vi "nPoints Concept - Pushbutton.vi"() -> ()   [LabVIEW 2013]
uses:
  <vilib>/Utility/error.llb/DialogType.ctl
  <vilib>/DAQmx/read.llb/DAQmx Read (Digital 1D Bool 1Chan 1Samp).vi
  <vilib>/DAQmx/create/channels.llb/DAQmx Create Channel (DI-Digital Input).vi
  <vilib>/DAQmx/miscellaneous.llb/DAQmx Fill In Error Info.vi
panel:
  out "Digital Data":i16(graph)
  in  "Line(s)":tag="Dev1/port0/line0:7"
  in  "Stop":bool
  out "Blank Button":bool
  # "Pushbutton Switch"
  # "5V"
  # "DIO"
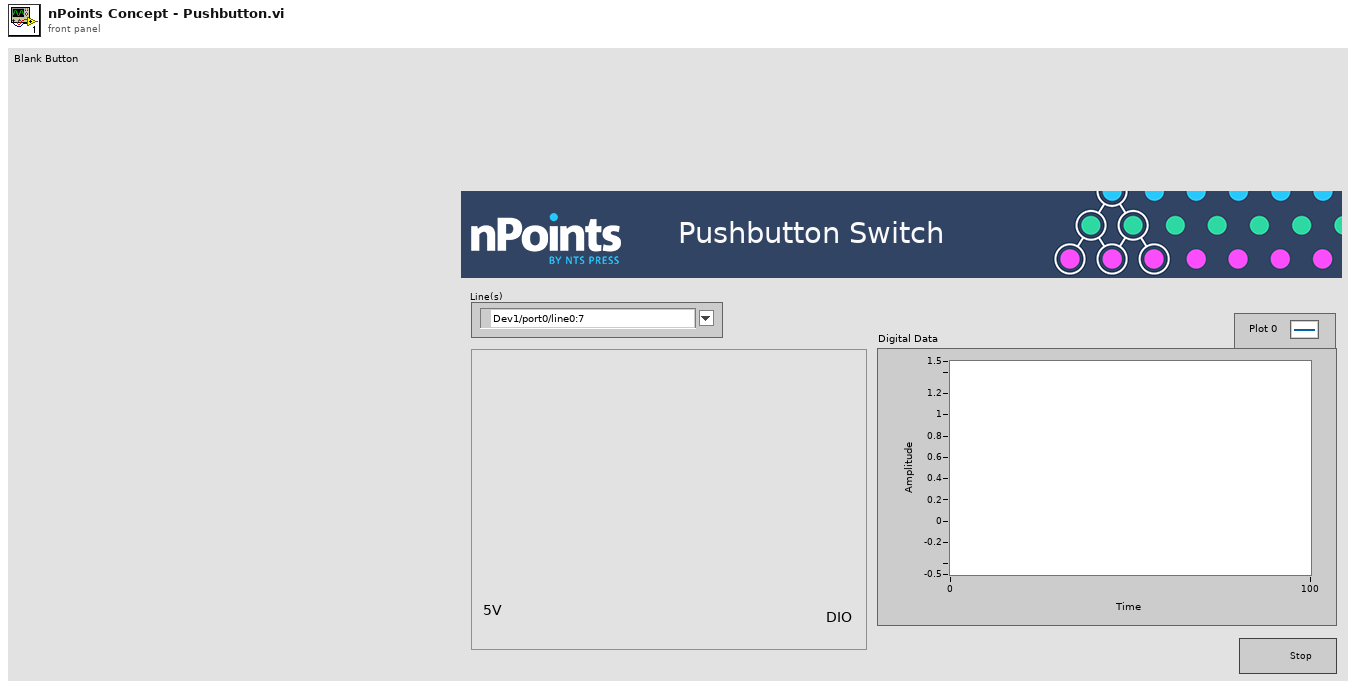
[diagram p1: front panel]
types:
  T1 = typedef "DialogType.ctl" = u16
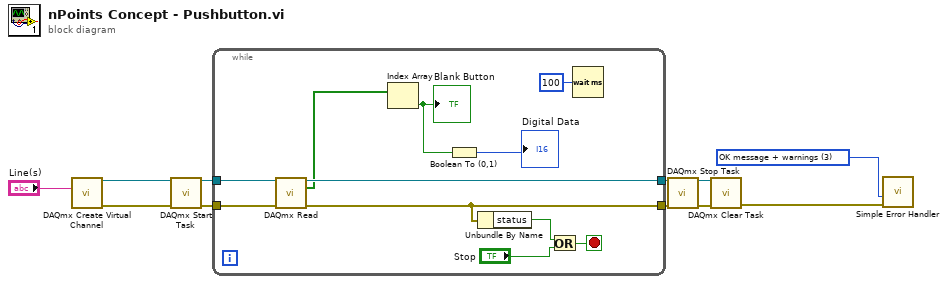
[diagram p0: block diagram]
diagram:
  w1 = T1 3 items=["no dialog", "OK message", "continue or stop message", "OK message + warnings", "continue/stop + warnings"] ("type of dialog (OK msg:1)")
  n1 = call-poly <vilib>:"DAQmx Create Virtual Channel.vi"("lines"="Line(s)") -> ("task out"=w6:refnum<k21>, "error out"=w7:errorcluster)  [unwired: 13 in]
  n2 = call <vilib>:"DAQmx Start Task.vi"("task/channels in"=w6, "error in"=w7) -> ("task out"=w11:refnum<k21>, "error out"=w10:errorcluster)  [unwired: 12 in]
  n3 = while {
    tunnel: w11 -> [w22]
    tunnel: w10 -> [w21]
    tunnel: [w18] -> w4
    tunnel: [w19] -> w5
    stop <- w20 stop-if-true
    n4 = call-poly <vilib>:"DAQmx Read.vi"("task/channels in"=w22, "error in"=w21) -> ("task out"=w19:refnum<k21>, "data"=w14:bool[], "error out"=w18:errorcluster)  [unwired: 11 in]
    n5 = Index Array(array=w14) -> (element=w13:bool)  [unwired: 1 in]
    "Blank Button" <- w13
    n6 = Boolean To (0,1)(Boolean=w13) -> (0, 1=→"Digital Data":i16)
    n7 = Unbundle By Name(w18) -> ("status"=w17:bool)
    n8 = Or(x=w17, y="Stop") -> (x .or. y?=w20:bool)
    n9 = Wait (ms)(milliseconds to wait=u32 100) -> ()  [unwired: 1 out]
  }
  n10 = call <vilib>:"DAQmx Stop Task.vi"("task/channels in"=w5, "error in"=w4) -> ("task out"=w3:refnum<k21>, "error out"=w2:errorcluster)  [unwired: 12 in]
  n11 = call <vilib>:"DAQmx Clear Task.vi"("task in"=w3, "error in"=w2) -> ("error out"=w9:errorcluster)  [unwired: 13 in]
  n12 = call <vilib>:"Simple Error Handler.vi"("type of dialog (OK msg:1)"=w1, "error in (no error)"=w9) -> ()  [unwired: 3 in, 5 out]
